vi "Configure Acquisition.vi"(0 "device session in":refnum<class "Device Session.lvclass">, 1 "pretrigger samples":u64, 2 "number of records is finite (T)":bool=TRUE, 5 "number of records":u64=1, 7 "number of samples":u64=1000, 9 "channels to store":u32[](array[numeric]), 11 "error in":errorcluster, 12 "additional configuration":T2={"record padding (samples)"=0, "require finite records to fit in memory"=TRUE, "timestamps per record"=1, "status fifo depth (records)"=10000}) -> (4 "device session out":refnum<class "Device Session.lvclass">, 6 "actual channels stored":bool[](array[boolean]), 8 "trigger Source":cluster{"Hi":bool, "Lo":bool}, 10 "TrigCfg 0":T1, 15 "error out":errorcluster)   [LabVIEW 2021, in "Device Session.lvclass"]
doc: "Configures the acquisition. You can specify which channels to acquire from, how many records to acquire, and how many samples to acquire. You must run this VI before running the <B>Initiate</B> VI.\n\n<B>Input Parameters</B>\n\n<B>device session in</B> is a reference to the Device Session object, which contains a session to each instrument design library used in this sample project. This parameter is obtained from the 'Open Session' VI.\n\n<B>number of records is finite (T)</B> specifies whether to acquire a finite number of records, or to acquire records continuously.\n\n<B>pretrigger samples</B> specifies, for every record, the minimum number of samples that must be stored from the time period immediately before the Reference Trigger occurred.\n\n<B>number of records</B> specifies the number of records to acquire. The default value is 1.\n\n<B>number of samples</B> specifies the number of samples to acquire. The default value is 1000.\n\n<B>channels to store</B> specifies the channels to store in memory. By default, only the channels configured using the 'Configure Channel' VI are stored.\n\n<B>additional configuration</B> specifies additional advanced configurations.\n\n<B>additional configuration.record padding (samples)</B> specifies additional padding to allocate for a record. This parameter can be useful in combination with adjusting the Reference Trigger position. The default value is 0.\n\n<B>additional configuration.require finite records to fit in memory</B> specifies that the requested number of records and samples must fit into memory for finite acquisitions. This parameter ensures that requested data cannot be overwritten for finite acquisitions. The default is TRUE.\n\n<B>additional configuration.timestamps per record</B> specifies the number of timestamp values the FPGA captures for each record. This value must match the number of timestamps per record provided to the Write VI of the Multirecord Acquisition FPGA library. The default value is 0.\n\n<B>additional configuration.status fifo depth (records)</B> Sets the depth of the record status DMA FIFO. The Status FIFO reports information about the current state of the acquisition to the host.\nEnsure that the Status FIFO is deep enough for the rate at which the host consumes this FIFO. If the Status FIFO is full, memory writes are delayed. Eventually, this can cause the Write FIFO to fill up and overflow. The host consumes the entire Status FIFO each time you fetch a record or query acquisition status. The value is specified in units of records. The default value is 10,000 records.\n\n<B>error in</B> describes error conditions that occur before this node runs. This input provides standard 'error in' functionality.\n\n<B>Output Parameters</B>\n\n<B>device session out</B> passes a reference to the session to the next VI.\n\n<B>actual channels stored</B> returns the number of channels stored as a power of two.\n\n<B>error out</B> contains error information. This output provides standard 'error out' functionality."
uses:
  Device Session.lvclass
  <instrlib>/_niInstr/Multirecord Acquisition/Interface/v1/Host/Public/Additional Acquisition Configuration.ctl
  Device Session.lvclass/Device Session.ctl
  <vilib>/Utility/error.llb/Error Cluster From Error Code.vi
  <vilib>/rvi/errors/niLvFpgaAdjustHostInterfaceError.vi
  <vilib>/rvi/interface/nirviReadWriteControl/nirviReadWriteControl.xnode
  FPGA Refnum.ctl
  <instrlib>/_niInstr/Multirecord Acquisition/Interface/v1/Host/niInstr Multirecord Acquisition v1 Host.lvclass
  <vilib>/rvi/interface/Simulation/niFpgaSimulationCallBeginRW.vi
  NiFpgaLv.dll
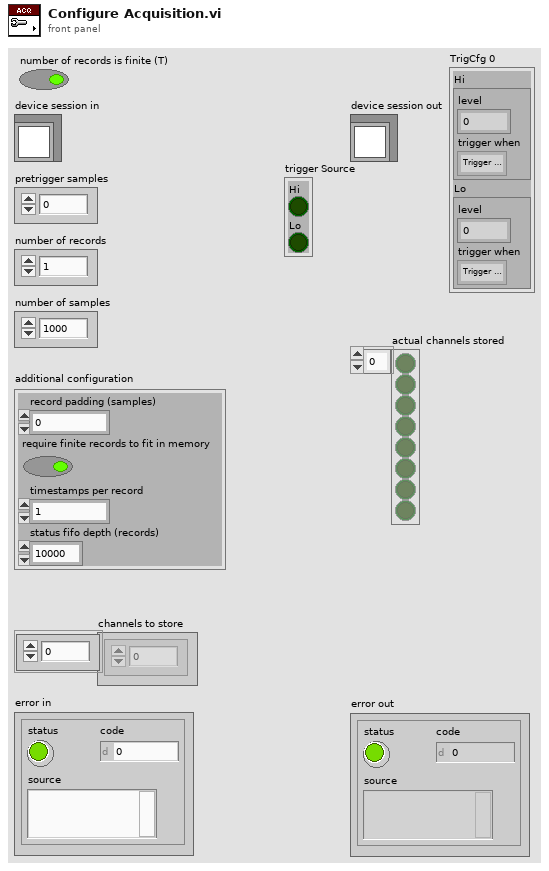
[diagram p1: front panel]
types:
  T1 = cluster{"Hi":cluster{"level":fxp<+/-,18,1>, "trigger when":enum8{"Trigger Above", "Trigger Below"}}, "Lo":cluster{"level":fxp<+/-,18,1>, "trigger when":enum8{"Trigger Above", "Trigger Below"}}}
  T2 = typedef "niInstr Multirecord Acquisition v1 Host.lvclass/Additional Acquisition Configuration.ctl" = cluster{"record padding (samples)":u64, "require finite records to fit in memory":bool, "timestamps per record":u32, "status fifo depth (records)":u32}
  T3 = typedef "Device Session.lvclass/Device Session Object.ctl" = cluster{"fpga reference":T4, "reg bus":refnum<class "niInstr FIFO Register Bus v1 Host.lvclass">, "subsystem map":refnum<class "niInstr Subsystem Map v1 Host.lvclass">, "cal data":refnum<class "niHSAI Cal Data v1 Host.lvclass">, "config":refnum<class "niHSAI Group A Config v1 Host.lvclass">, "acquisition":refnum<class "niInstr Multirecord Acquisition v1 Host.lvclass">, "number of selected acq channels":u8, "selected acq channels":bool[], "number of channels":u32, "configured channels":bool[], "acq configuration":cluster{"number of samples":u64, "number of records":u64, "pretrigger samples":u64}, "actual channel configuration":T5[], "sample clock rate (Hz)":dbl, "scaling coefficients":T9[]}
  T4 = typedef "Device Session.lvclass/FPGA Refnum.ctl" = refnum<k20>
  T5 = typedef "niHSAI Types v1 Host.lvlib/Channel Configuration.ctl" = cluster{"channel":u32, "coupling":T6, "impedance":T7, "bandwidth":T8, "vertical range":dbl, "vertical offset":dbl}
  T6 = typedef "niHSAI Types v1 Host.lvlib/Coupling.ctl" = enum8{"Default", "DC", "AC"}
  T7 = typedef "niHSAI Types v1 Host.lvlib/Impedance.ctl" = enum8{"Default", "1 mega ohm", "50 ohm"}
  T8 = typedef "niHSAI Types v1 Host.lvlib/Bandwidth.ctl" = enum8{"Default", "Full Bandwidth", "Anti-alias Filter", "150 MHz"}
  T9 = typedef "niInstr Multirecord Acquisition v1 Host.lvclass/Scaling Coefficient.ctl" = cluster{"gain":dbl, "offset":dbl}
  T10 = cluster{"Hi":cluster{"level":fxp<+/-,18,5>, "trigger when":enum8{"Trigger Above", "Trigger Below"}}, "Lo":cluster{"level":fxp<+/-,18,5>, "trigger when":enum8{"Trigger Above", "Trigger Below"}}}
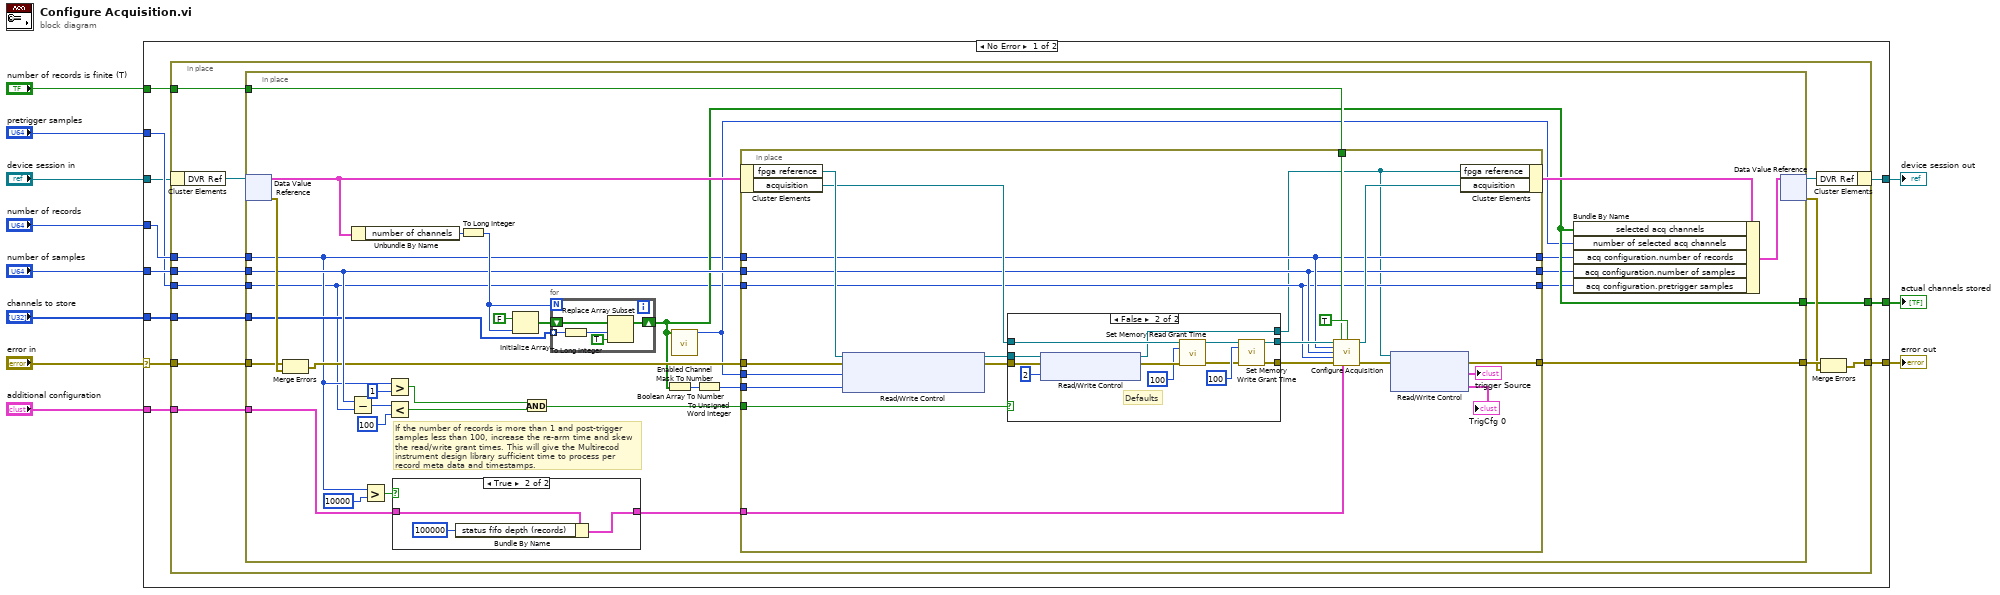
[diagram p0: block diagram]
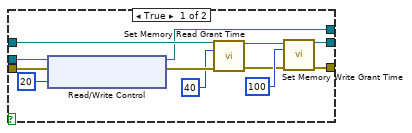
[diagram p2: hidden frame]
diagram:
  n1 = case shown="No Error" "error in" {
    selector: "error in" -> [w22 w125]
    tunnel: [w14 w125] -> w10
    tunnel: "device session in" -> [w12 w124]
    tunnel: [w13 w124] -> w8
    tunnel: "number of records" -> [w21 _]
    tunnel: "number of samples" -> [w20 _]
    tunnel: "channels to store" -> [w19 _]
    tunnel: [w18 _] -> w4
    tunnel: "pretrigger samples" -> [w17 _]
    tunnel: "additional configuration" -> [w16 _]
    tunnel: "number of records is finite (T)" -> [w15 _]
    frame No Error {
      n2 = in-place {
        in-place-border: w22 -> [w35]
        in-place-border: w21 -> [w34]
        in-place-border: w20 -> [w33]
        in-place-border: w19 -> [w30]
        in-place-border: [w29] -> w18
        in-place-border: w17 -> [w28]
        in-place-border: w16 -> [w27]
        in-place-border: w15 -> [w26]
        in-place-border: [w25] -> w14
        n3 = in-place-cluster #1(w12) -> ("DVR Ref"=w24:refnum<data-value>)
        n4 = in-place {
          in-place-border: w35 -> [w63]
          in-place-border: [w66] -> w32
          in-place-border: w34 -> [w37]
          in-place-border: w33 -> [w49]
          in-place-border: w30 -> [w38]
          in-place-border: [w43] -> w29
          in-place-border: w28 -> [w36]
          in-place-border: w27 -> [w47]
          in-place-border: w26 -> [w60]
          # "If the number of records is more than 1 and post-trigger samples less than 100, increase the re-arm time and skew the read/write grant times. This will give the Multirecod instrument design library sufficient time to process per record meta data and timestamps."
          n5 = in-place-dvr #2(w24) -> (w45:T3, w67:errorcluster)
          n6 = Merge Errors(w63, w67) -> (w48:errorcluster)
          n7 = Subtract(x=w49, y=w36) -> (x-y=w57:u64)
          n8 = Unbundle By Name(w45) -> ("number of channels"=w59:u32)
          n9 = Greater?(x=w37, y=u64 10000) -> (0:w50:bool)
          n10 = Greater?(x=w37, y=u64 1) -> (0:w54:bool)
          n11 = Less?(x=w57, y=u64 100) -> (x < y?=w53:bool)
          n12 = case shown="True" w50 {
            tunnel: w47 -> [w115 w118]
            tunnel: [w115 w116] -> w46
            frame False {
            }
            frame True {
              n13 = Bundle By Name(cluster=w118, "status fifo depth (records)"=u32 100000) -> (w116:T2)
            }
          }
          n14 = To Long Integer(number=w59) -> (32bit integer=w58:i32)
          n15 = Initialize Array(FALSE, w58) -> (w61:bool[])
          n16 = And(x=w54, y=w53) -> (x .and. y?=w52:bool)
          n17 = for {
            N: w58 -> [_]
            tunnel: w38 -> [w120] mode=indexing
            shift-right: [w122] -> w43
            shift-left: w61 -> [w121]
            n18 = To Long Integer(number=w120) -> (32bit integer=w119:i32)
            n19 = Replace Array Subset(array=w121, new element=TRUE ("new element/subarray"), index=w119) -> (w122:bool[])
          }
          n20 = Boolean Array To Number(Boolean array=w43) -> (number=w65:u32)
          n21 = call "Enabled Channel Mask To Number.vi"("selected acquisition channels to store"=w43) -> ("number of selected channels"=w42:u8)  [unwired: 14 in]
          n22 = To Unsigned Word Integer(number=w65) -> (unsigned 16bit integer=w64:u16)
          n23 = in-place {
            in-place-border: [w72] -> w66
            in-place-border: w64 -> [w90]
            in-place-border: w60 -> [w88]
            in-place-border: w52 -> [w83]
            in-place-border: w36 -> [w74]
            in-place-border: w49 -> [w75]
            in-place-border: w48 -> [w82]
            in-place-border: w37 -> [w76]
            in-place-border: w42 -> [w81]
            in-place-border: w46 -> [w80]
            in-place-border: [w76] -> w41
            in-place-border: [w75] -> w40
            in-place-border: [w74] -> w39
            n24 = in-place-cluster #3(w45) -> ("fpga reference"=w79:T4, "acquisition"=w78:refnum<class "niInstr Multirecord Acquisition v1 Host.lvclass">)
            n25 = xnode "Read/Write Control"("FPGA VI Reference In"=w79, "error in"=w82, "channel.number of channels"=w81, "channel.enable mask"=w90) -> ("FPGA VI Reference Out"=w87:T4, "error out"=w86:errorcluster)
            n26 = case shown="False" w83 {
              tunnel: w78 -> [w96 w108]
              tunnel: w87 -> [w97 w109]
              tunnel: w86 -> [w95 w107]
              tunnel: [w94 w106] -> w85
              tunnel: [w93 w105] -> w84
              tunnel: [w91 w103] -> w71
              frame True {
                n27 = xnode "Read/Write Control"("FPGA VI Reference In"=w97, "error in"=w95, "trigger.rearm delay"=u16 20 ("trigger.rearm time")) -> ("FPGA VI Reference Out"=w91:T4, "error out"=w102:errorcluster)
                n28 = call-dynamic "Set Memory Read Grant Time.vi"("session in"=w96, "grant time (clocks)"=u32 40, "error in"=w102) -> ("session out"=w98:refnum<class "niInstr Multirecord Acquisition v1 Host.lvclass">, "error out"=w99:errorcluster)  [unwired: 11 in]
                n29 = call-dynamic "Set Memory Write Grant Time.vi"("session in"=w98, "grant time (clocks)"=u32 100, "error in"=w99) -> ("session out"=w93:refnum<class "niInstr Multirecord Acquisition v1 Host.lvclass">, "error out"=w94:errorcluster)  [unwired: 11 in]
              }
              frame False {
                # "Defaults"
                n30 = xnode "Read/Write Control"("FPGA VI Reference In"=w109, "error in"=w107, "trigger.rearm delay"=u16 2 ("trigger.rearm time")) -> ("FPGA VI Reference Out"=w103:T4, "error out"=w114:errorcluster)
                n31 = call-dynamic "Set Memory Read Grant Time.vi"("session in"=w108, "grant time (clocks)"=u32 100, "error in"=w114) -> ("session out"=w110:refnum<class "niInstr Multirecord Acquisition v1 Host.lvclass">, "error out"=w111:errorcluster)  [unwired: 11 in]
                n32 = call-dynamic "Set Memory Write Grant Time.vi"("session in"=w110, "grant time (clocks)"=u32 100, "error in"=w111) -> ("session out"=w105:refnum<class "niInstr Multirecord Acquisition v1 Host.lvclass">, "error out"=w106:errorcluster)  [unwired: 11 in]
              }
            }
            n33 = call-dynamic "Configure Acquisition.vi"("session in"=w84, "number of records is finite"=w88, "number of samples is finite"=TRUE, "number of records"=w76, "number of samples"=w75, "pretrigger samples"=w74, "error in"=w85, "additional acquisition configuration"=w80) -> ("session out"=w77:refnum<class "niInstr Multirecord Acquisition v1 Host.lvclass">, "error out"=w73:errorcluster)  [unwired: 5 in, 1 out]
            n34 = xnode "Read/Write Control"("FPGA VI Reference In"=w71, "error in"=w73) -> ("error out"=w72:errorcluster, "trigger Source"=→"trigger Source":cluster{"Hi":bool, "Lo":bool}, "TrigCfg 0"=→"TrigCfg 0":T10)  [unwired: 1 out]
            n35 = in-place-cluster #3("fpga reference"=w71, "acquisition"=w77) -> (w44:T3)
          }
          n36 = Bundle By Name(cluster=w44, "selected acq channels"=w43, "number of selected acq channels"=w42, "acq configuration.number of records"=w41, "acq configuration.number of samples"=w40, "acq configuration.pretrigger samples"=w39) -> (w68:T3)
          n37 = in-place-dvr #2(w68) -> (w23:refnum<data-value>, w31:errorcluster)
        }
        n38 = in-place-cluster #1("DVR Ref"=w23) -> (w13:refnum<class "Device Session.lvclass">)
        n39 = Merge Errors(w32, w31) -> (w25:errorcluster)
      }
    }
    frame Error {
    }
  }
  "error out" <- w10
  "device session out" <- w8
  "actual channels stored" <- w4
